vi "getDposInCurrentUnits.vi"(8 "error in (no error)":errorcluster, 11 "Axis in":refnum<class "Axis.lvclass">) -> (0 "error out":errorcluster, 2 "DPOS In Current Units":dbl, 3 "Axis out":refnum<class "Axis.lvclass">)   [LabVIEW 2019, in "Axis.lvclass"]
uses:
  Axis.lvclass
  Axis.lvclass/Axis.ctl
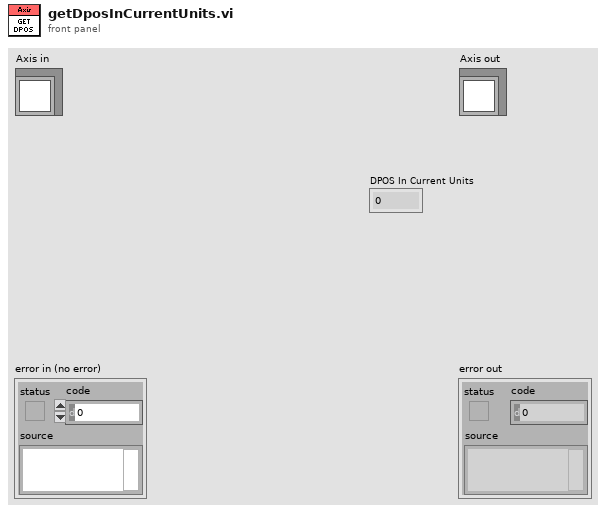
[diagram p1: front panel]
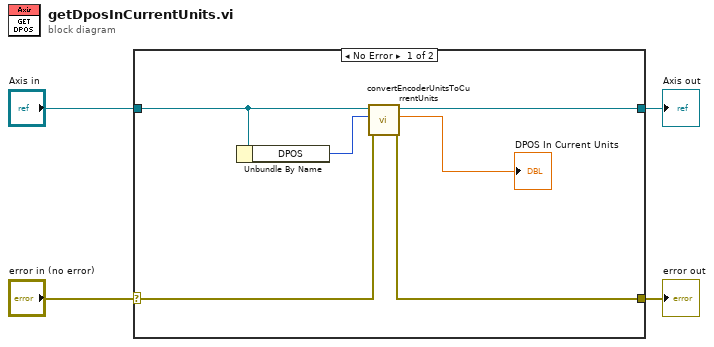
[diagram p0: block diagram]
diagram:
  n1 = case shown="No Error" "error in (no error)" {
    selector: "error in (no error)" -> [w8 w12]
    tunnel: [w9 w11] -> w2
    tunnel: "Axis in" -> [w10 w11]
    tunnel: [w7 w12] -> w1
    frame No Error {
      n2 = Unbundle By Name(w10) -> ("DPOS"=w6:i32)
      n3 = call-dynamic "convertEncoderUnitsToCurrentUnits.vi"("error in (no error)"=w8, "Value In Encoder Units"=w6, "Axis in"=w10) -> ("error out"=w7:errorcluster, "Value In Current Units"=→"DPOS In Current Units":dbl, "Axis out"=w9:refnum<class "Axis.lvclass">)  [unwired: 6 in]
    }
    frame Error {
    }
  }
  "error out" <- w1
  "Axis out" <- w2
